vi "Generate and Save Method VIs.vi"(7 "Template VI Dir":path, 9 "Class Param Writer":refnum<class "Abstract Param Writer.lvclass">, 10 "Class Info":T1[](array[typedef]), 11 "Module Class Ref Map":variant) -> (3 "Reduced Module Class Ref Map":variant)   [LabVIEW 2013]
doc: "Copyright (c) 2016 Sze Howe Koh\n\nThis Source Code Form is subject to the terms of the Mozilla Public License, v. 2.0. If a copy of the MPL was not distributed with this file, You can obtain one at http://mozilla.org/MPL/2.0/."
uses:
  Param Writers/Abstract Param Writer/Abstract Param Writer.lvclass
  Data Structures/JSON/Class.ctl
  Data Structures/JSON/Enum.ctl
  Data Structures/JSON/Enum Value.ctl
  Data Structures/JSON/Method.ctl
  Data Structures/JSON/Param.ctl
  Data Structures/JSON/Connector Pane.ctl
  Data Structures/JSON/Connector Pane Terminal.ctl
  Data Structures/JSON/Property.ctl
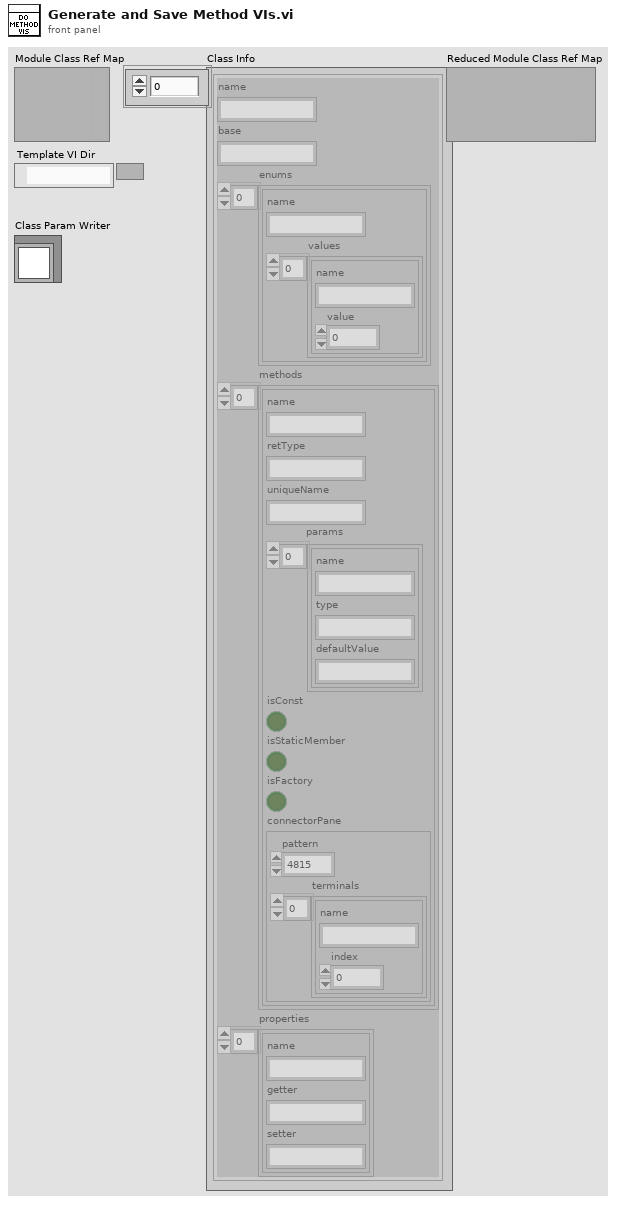
[diagram p1: front panel]
types:
  T1 = typedef "Class.ctl" = cluster{"name":string, "base":string, "enums":T2[], "methods":T4[], "properties":T8[]}
  T2 = typedef "Enum.ctl" = cluster{"name":string, "values":T3[]}
  T3 = typedef "Enum Value.ctl" = cluster{"name":string, "value":i32}
  T4 = typedef "Method.ctl" = cluster{"name":string, "retType":string, "uniqueName":string, "params":T5[], "isConst":bool, "isStaticMember":bool, "isFactory":bool, "connectorPane":T6}
  T5 = typedef "Param.ctl" = cluster{"name":string, "type":string, "defaultValue":string}
  T6 = typedef "Connector Pane.ctl" = cluster{"pattern":u32, "terminals":T7[]}
  T7 = typedef "Connector Pane Terminal.ctl" = cluster{"name":string, "index":u32}
  T8 = typedef "Property.ctl" = cluster{"name":string, "getter":string, "setter":string}
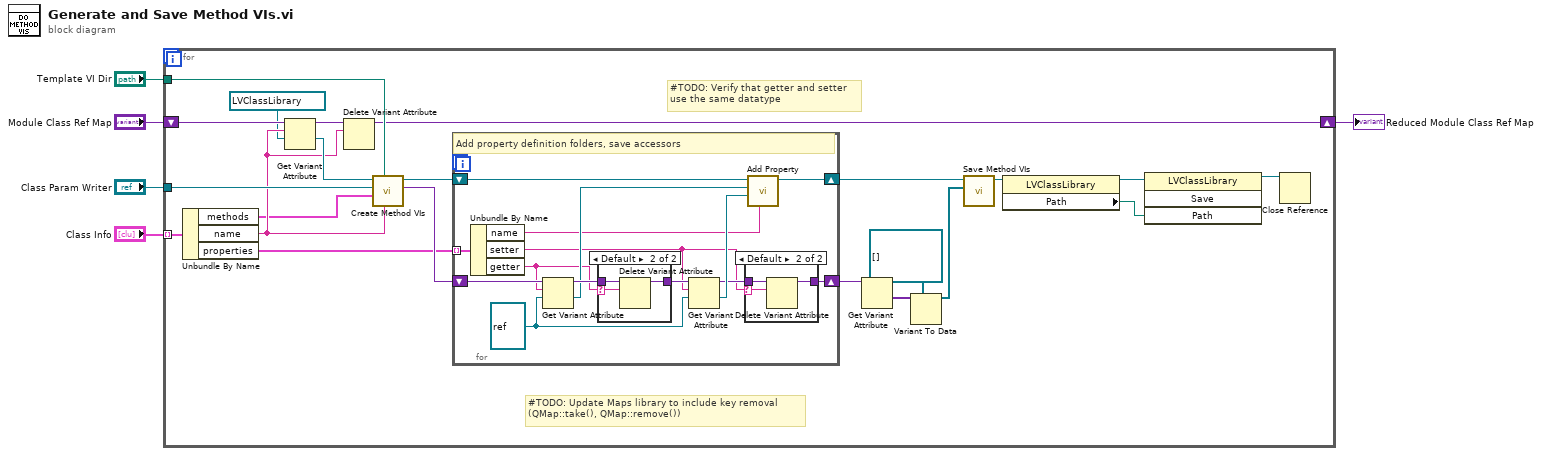
[diagram p0: block diagram]
diagram:
  n1 = for {
    tunnel: "Template VI Dir" -> [w16]
    tunnel: "Class Param Writer" -> [w15]
    tunnel: "Class Info" -> [w14] mode=indexing
    shift-right: [w8] -> w1
    shift-left: "Module Class Ref Map" -> [w13]
    # "#TODO: Verify that getter and setter\nuse the same datatype"
    # "#TODO: Update Maps library to include key removal\n(QMap::take(), QMap::remove())"
    n2 = Unbundle By Name(w14) -> ("methods"=w10:T4[], "name"=w11:string, "properties"=w21:T8[])
    n3 = Get Variant Attribute(Variant=w13, name=w11, default value (empty Variant)=refnum<vi> refnum ("QObject")) -> (duplicate Variant=w6:variant, value=w12:refnum<vi>)  [unwired: 1 in, 2 out]
    n4 = Delete Variant Attribute(6:w11, 7:w6) -> (3:w8:variant)  [unwired: 1 in, 2 out]
    n5 = call "Create Method VIs.vi"("Projection Source Name"=w11, "Template VI Dir"=w16, "Methods"=w10, "Class Param Writer"=w15, "Class"=w12) -> ("Method Ref Map"=w22:variant, "Class Dup"=w23:refnum<vi>)  [unwired: 5 in]
    n6 = for {
      shift-right: [w40] -> w24
      shift-left: w23 -> [w41]
      shift-right: [w29] -> w27
      shift-left: w22 -> [w39]
      tunnel: w21 -> [w33] mode=indexing
      w34 = refnum<vi> refnum ("reference out")
      # "Add property definition folders, save accessors"
      n7 = Unbundle By Name(w33) -> ("name"=w32:string, "setter"=w28:string, "getter"=w31:string)
      n8 = Get Variant Attribute(Variant=w39, name=w31, default value (empty Variant)=w34) -> (duplicate Variant=w38:variant, value=w37:refnum<vi>)  [unwired: 1 in, 2 out]
      n9 = case shown="Default" w31 {
        selector: w31 -> [_ w47]
        tunnel: w38 -> [w46 w49]
        tunnel: [w46 w48] -> w36
        frame "" {
        }
        frame Default {
          n10 = Delete Variant Attribute(6:w47, 7:w49) -> (3:w48:variant)  [unwired: 1 in, 2 out]
        }
      }
      n11 = Get Variant Attribute(Variant=w36, name=w28, default value (empty Variant)=w34) -> (duplicate Variant=w30:variant, value=w35:refnum<vi>)  [unwired: 1 in, 2 out]
      n12 = case shown="Default" w28 {
        selector: w28 -> [_ w43]
        tunnel: w30 -> [w42 w45]
        tunnel: [w42 w44] -> w29
        frame "" {
        }
        frame Default {
          n13 = Delete Variant Attribute(6:w43, 7:w45) -> (3:w44:variant)  [unwired: 1 in, 2 out]
        }
      }
      n14 = call "Add Property.vi"("Property Name"=w32, "Setter"=w35, "Getter"=w37, "Class"=w41) -> ("Class Dup"=w40:refnum<vi>)  [unwired: 7 in]
    }
    n15 = Get Variant Attribute(Variant=w27) -> (values=w26:variant[])  [unwired: 3 in, 3 out]
    n16 = Variant To Data(type=refnum<vi>[] [], Variant=w26) -> (data=w17:refnum<vi>[])  [unwired: 1 in, 1 out]
    n17 = call "Save Method VIs.vi"("Class Methods"=w17, "LVClass"=w24) -> ("LVClass Dup"=w20:refnum<vi>)  [unwired: 9 in]
    n18 = property class="LVClassLibrary"(reference=w20) -> (reference out=w19:refnum<vi>, "Path"=w18:path)  [unwired: 1 in, 1 out]
    n19 = invoke class="LVClassLibrary" method="Save"(reference=w19, "Path"=w18) -> (reference out=w9:refnum<vi>)  [unwired: 2 in, 3 out]
    n20 = Close Reference(reference=w9) -> ()  [unwired: 1 in, 1 out]
  }
  "Reduced Module Class Ref Map" <- w1
